vi "XL320_Move Motor.vi"(0 "VISA resource name":refnum<visa-resource-name>, 5 "Motor ID (0)":u8, 7 "Goal Position (150 deg)":dbl=150.0, 9 "Goal Speed (RPM)":dbl, 11 "error in (no error)":errorcluster) -> (4 "VISA resource name out":refnum<visa-resource-name>, 6 "Command to Serial":string, 15 "error out":errorcluster)   [LabVIEW 2017, in "Dynamixel XL320.lvlib"]
doc: "Sets the goal position for the motor."
uses:
  <instrlib>/Dynamixel XL320 (Drivers instrument)/Dynamixel XL320.lvlib
  <instrlib>/Dynamixel XL320 (Drivers instrument)/Public/Configure/XL320_Select_Action.ctl
panel:
  # "Ghislain REMY, IUT de Cachan, 2015 December 2015"
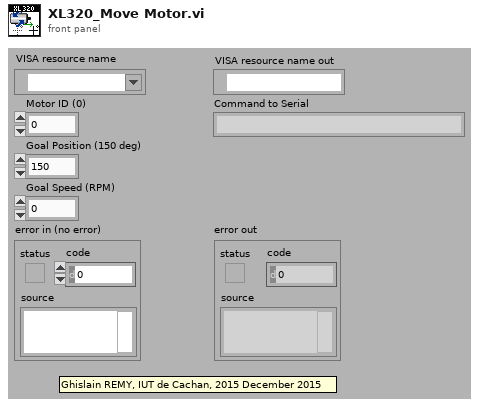
[diagram p1: front panel]
types:
  T1 = enum16{"big-endian, network order", "native, host order", "little-endian"}
  T2 = typedef "Dynamixel XL320.lvlib/XL320_Select_Action.ctl" = u8
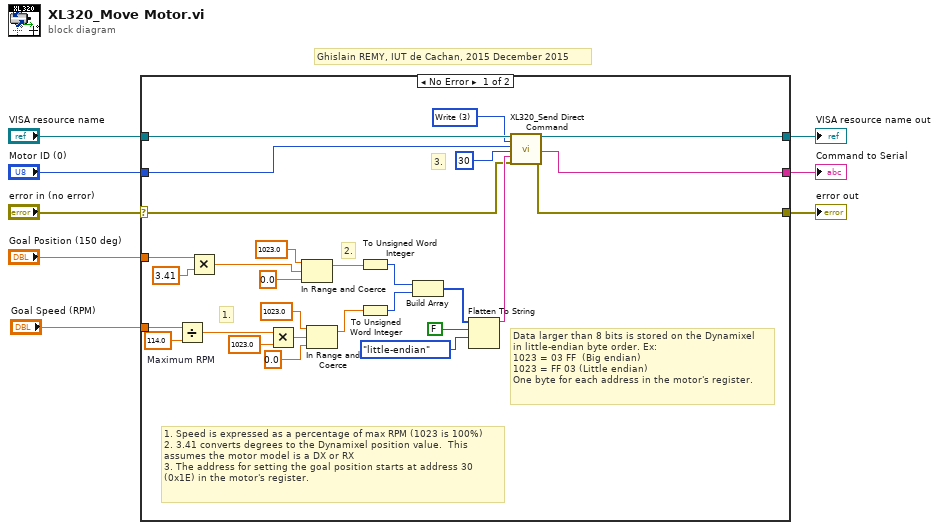
[diagram p0: block diagram]
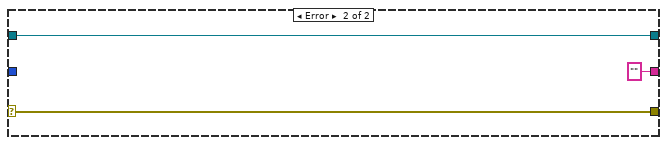
[diagram p2: hidden frame]
diagram:
  # "Ghislain REMY, IUT de Cachan, 2015 December 2015"
  n1 = case shown="No Error" "error in (no error)" {
    selector: "error in (no error)" -> [w13 w39]
    tunnel: "VISA resource name" -> [w17 w38]
    tunnel: [w11 w38] -> w7
    tunnel: [w12 w39] -> w6
    tunnel: "Motor ID (0)" -> [w16 _]
    tunnel: "Goal Position (150 deg)" -> [w32 _]
    tunnel: "Goal Speed (RPM)" -> [w31 _]
    tunnel: [w10 "" ("Command to Serial")] -> w1
    frame No Error {
      w9 = T2 3 items=["Ping"=1, "Read"=2, "Write"=3, "Registered Write"=4, "Action"=5, "Reset"=6, "Reboot"=8, "Status"=85, "Sync Read"=130, "Sync Write"=131, "Bulk Read"=146, "Bulk Write"=147] ("Select Action")
      w28 = 114.0  # Maximum RPM
      # "3."
      # "2."
      # "1."
      # "Data larger than 8 bits is stored on the Dynamixel \nin little-endian byte order. Ex:\n1023 = 03 FF  (Big endian)\n1023 = FF 03 (Little endian)\nOne byte for each address in the motor's register."
      # "1. Speed is expressed as a percentage of max RPM (1023 is 100%)\n2. 3.41 converts degrees to the Dynamixel position value.  This \nassumes the motor model is a DX or RX\n3. The address for setting the goal position starts at address 30\n(0x1E) in the motor's register."
      n2 = Divide(x=w31, y=w28) -> (x/y=w30:dbl)
      n3 = Multiply(x=w32, y=3.41) -> (x*y=w18:dbl)
      n4 = Multiply(x=w30, y=1023.0 ("upper limit")) -> (x*y=w35:dbl)
      n5 = In Range and Coerce(upper limit=1023.0, x=w18, lower limit=0.0) -> (coerced(x)=w19:dbl)  [unwired: 1 out]
      n6 = In Range and Coerce(upper limit=1023.0, x=w35, lower limit=0.0) -> (coerced(x)=w22:dbl)  [unwired: 1 out]
      n7 = To Unsigned Word Integer(number=w19) -> (unsigned 16bit integer=w25:u16)
      n8 = To Unsigned Word Integer(number=w22) -> (unsigned 16bit integer=w24:u16)
      n9 = Build Array(w25, w24) -> (w23:u16[])
      n10 = Flatten To String(anything=w23, prepend array or string size? (T)=FALSE, byte order (0:big-endian, network order)=T1."little-endian") -> (data string=w14:string)  [unwired: 1 in, 2 out]
      n11 = call <instrlib>:"XL320_Send Direct Command.vi"("VISA resource name"=w17, "Select Action"=w9, "Motor ID (0)"=w16, "Address"=u16 30, "Parameters"=w14, "Error in (no error)"=w13) -> ("VISA resource name out"=w11:refnum<visa-resource-name>, "Command to Serial"=w10:string, "Error out"=w12:errorcluster)  [unwired: 11 in]
    }
    frame Error {
    }
  }
  "VISA resource name out" <- w7
  "error out" <- w6
  "Command to Serial" <- w1
